vi "Chip Selection to Boolean.vi"(11 "chip select":enum16{"1st chip", "2nd chip"}(ring)) -> (3 "E?E1:E2":bool=TRUE)   [LabVIEW 2015, in "HD44780 FPGA.lvlib"]
uses:
  <vilib>/EmbeddedDisplay/Hitachi HD44780/FPGA/HD44780 FPGA.lvlib
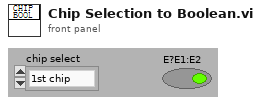
[diagram p1: front panel]
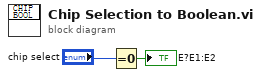
[diagram p0: block diagram]
diagram:
  n1 = Equal To 0?(x="chip select") -> (x = 0?=→"E?E1:E2":bool)
